vi "RobotLiftSubsystem.vi"   [LabVIEW 2017]
uses:
  RobotLiftCommand.ctl
  RunMode.ctl
  RobotLiftOutput.ctl
  RobotSubsystem.lvclass
  SubsystemData/RobotLiftData/RobotLiftData.lvclass
  Subsystem/Subsystem.lvclass
  SubsystemData/RobotLiftData/RobotLift.lvclass
panel:
  # "This is responsable for controling the jacks"
types:
  T1 = typedef "RobotLiftData.lvclass/RobotLiftOutput.ctl" = cluster{"LeftRobotLiftSetting":dbl, "RightRobotLiftSetting":dbl, "RampReleaseSetting":bool}
  T2 = typedef "RobotLiftData.lvclass/RobotLiftCommand.ctl" = cluster{"Left Lift":cluster{"Up":bool, "Down":bool}, "Right Lift":cluster{"Up":bool, "Down":bool}, "Release Ramps":bool, "Mode":T3}
  T3 = typedef "RobotSubsystem.lvclass/RunMode.ctl" = enum16{"Auto", "Teleop", "Disabled"}
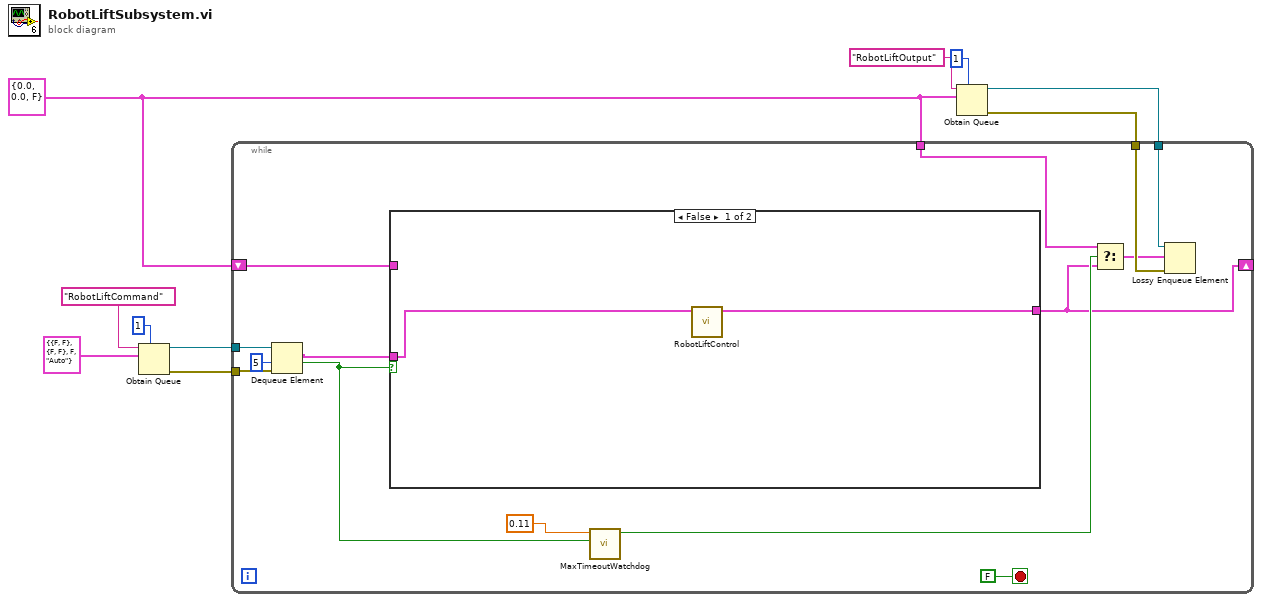
[diagram p0: block diagram]
diagram:
  w1 = T1 {"LeftRobotLiftSetting"=0.0, "RightRobotLiftSetting"=0.0, "RampReleaseSetting"=FALSE} ("RobotLiftOutput")
  n1 = Obtain Queue(max queue size (-1, unlimited)=1, name (unnamed)="RobotLiftCommand", element data type=T2 {"Left Lift"={"Up"=FALSE, "Down"=FALSE}, "Right Lift"={"Up"=FALSE, "Down"=FALSE}, "Release Ramps"=FALSE, "Mode"=enum."Auto"} ("Robot Lift Command")) -> (queue out=w7:refnum<queue>, error out=w6:errorcluster)  [unwired: 2 in, 1 out]
  n2 = Obtain Queue(max queue size (-1, unlimited)=1, name (unnamed)="RobotLiftOutput", element data type=w1) -> (queue out=w3:refnum<queue>, error out=w2:errorcluster)  [unwired: 2 in, 1 out]
  n3 = while {
    tunnel: w7 -> [w22]
    tunnel: w6 -> [w23]
    tunnel: w3 -> [w17]
    tunnel: w2 -> [w16]
    tunnel: w1 -> [w11]
    shift-right: [w13] -> _
    shift-left: w1 -> [w12]
    stop <- FALSE stop-if-true
    n4 = Dequeue Element(queue=w22, timeout in ms (-1)=5, error in (no error)=w23) -> (element=w18:T2, timed out?=w20:bool)  [unwired: 2 out]
    n5 = case shown="False" w20 {
      tunnel: w18 -> [w25 _]
      tunnel: [w26 w27] -> w13
      tunnel: w12 -> [_ w27]
      frame False {
        n6 = call "RobotLiftControl.vi"("Robot Lift Command"=w25) -> ("RobotLiftOutput out"=w26:T1)  [unwired: 10 in]
      }
      frame True {
      }
    }
    n7 = call "MaxTimeoutWatchdog.vi"("Keep counting?"=w20, "Max Timeout (s)"=0.11 ("Time Target (s)")) -> ("Over Max Timeout?"=w15:bool)  [unwired: 9 in]
    n8 = Select(t=w11, s=w15, f=w13) -> (s? t:f=w14:T1)
    n9 = Lossy Enqueue Element(queue=w17, element=w14, error in (no error)=w16) -> ()  [unwired: 4 out]
  }
